vi "Package Version.vi"(8 "error in (no error)":errorcluster, 11 "GitPackage in":refnum<class "GitPackage.lvclass">) -> (0 "error out":errorcluster, 2 "Version":string)   [LabVIEW 2020, in "GPack.lvlib" / "GitPackage.lvclass"]
uses:
  GitPackage.lvclass
  GitPackage.lvclass/GitPackage.ctl
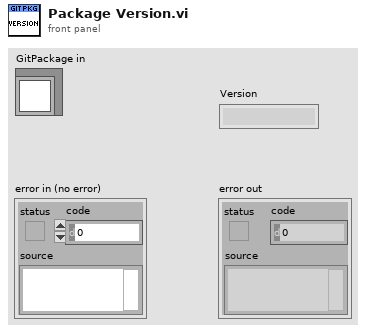
[diagram p1: front panel]
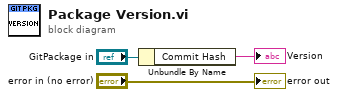
[diagram p0: block diagram]
diagram:
  n1 = Unbundle By Name("GitPackage in") -> ("Commit Hash"=→"Version":string)
  "error out" <- "error in (no error)"
